vi "Main_VirtualAccelerometer.vi"() -> ()   [LabVIEW 2019]
panel:
  out "Pos RSQ":dbl
  out "Original Pos versus Accelerometer Double Integration":cluster{i32[], dbl[]}(graph)
  out "V. Accel":dbl(graph)
  out "Mouse X Abs":i32
  in  "b":dbl=0.005 format="%#_13g"
  in  "m":dbl=0.001 format="%#_13g"
  in  "k":dbl=2000.0 format="%#_13g"
  out "Spring and Mass Position":cluster{"Mouse X Abs":i32, "yk":dbl}[](graph)
  out "Spring and Mass Position":cluster{"Mouse X Abs":i32, "yk":dbl}(graph)
  in  "stop":bool
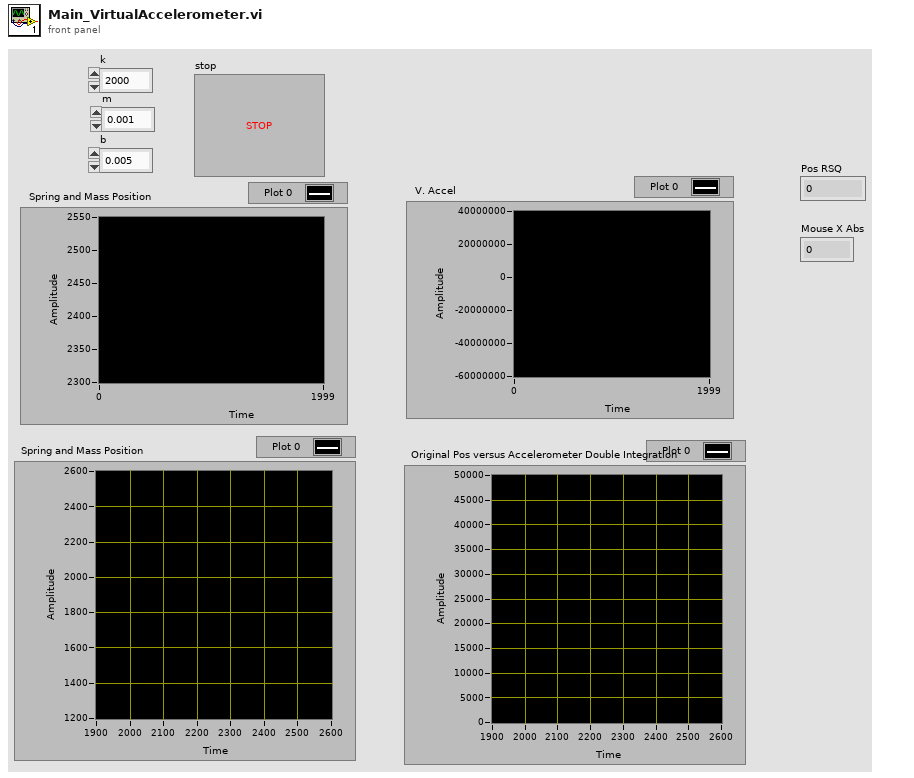
[diagram p1: front panel]
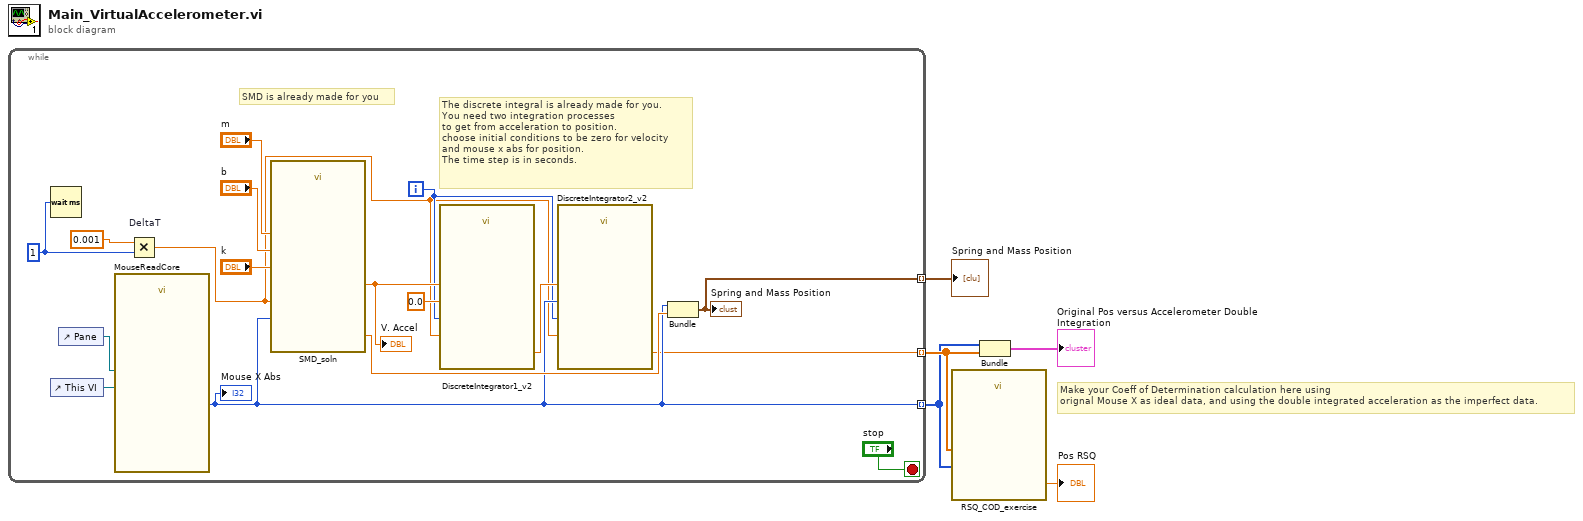
[diagram p0: block diagram]
diagram:
  # "Make your Coeff of Determination calculation here using\norignal Mouse X as ideal data, and using the double integrated acceleration as the imperfect data."
  n1 = while {
    tunnel: [w19] -> w5 mode=indexing
    tunnel: [w9] -> w1 mode=indexing
    tunnel: [w6] -> w2 mode=indexing
    i -> [w8]
    stop <- "stop" stop-if-true
    w13 = u32 1 ("milliseconds to wait")
    # "The discrete integral is already made for you.\nYou need two integration processes\nto get from acceleration to position.\nchoose initial conditions to be zero for velocity \nand mouse x abs for position.\nThe time step is in seconds."
    # "SMD is already made for you"
    n2 = Wait (ms)(milliseconds to wait=w13) -> ()  [unwired: 1 out]
    n3 = control-ref of="This VI"() -> (w21:refnum<vi>)
    n4 = control-ref of="Pane"() -> (w20:refnum<vi>)
    n5 = call "MouseReadCore.vi"("Pane"=w20, "VI in"=w21) -> ("Mouse X Abs"=w9:i32)  [unwired: 4 in, 5 out]
    "Mouse X Abs" <- w9
    n6 = Multiply "DeltaT"(x=0.001, y=w13) -> (x*y=w7:dbl)
    n7 = call "SMD_soln.vi"("k"="k", "b"="b", "m"="m", "Time Step"=w7, "xk"=w9) -> ("yk"=w15:dbl, "Accel"=w11:dbl)  [unwired: 5 in]
    "V. Accel" <- w11
    n8 = call "DiscreteIntegrator1_v2.vi"("Loop Iteration"=w8, "IC"=0.0, "Time Step"=w7, "Data in"=w11) -> ("Integ. Signal"=w10:dbl)  [unwired: 7 in]
    n9 = call "DiscreteIntegrator2_v2.vi"("Loop Iteration"=w8, "IC"=w9, "Time Step"=w7, "Data in"=w10) -> ("Integ. Signal"=w6:dbl)  [unwired: 7 in]
    n10 = Bundle("Mouse X Abs"=w9, "yk"=w15) -> (w19:cluster{"Mouse X Abs":i32, "yk":dbl})  [unwired: 1 in]
    "Spring and Mass Position" <- w19
  }
  "Spring and Mass Position" <- w5
  n11 = call "RSQ_COD_exercise.vi"("Data Yi's"=w2, "Model fi's"=w1) -> ("COD-RSQ"=→"Pos RSQ":dbl)  [unwired: 9 in]
  n12 = Bundle(w1, w2) -> (→"Original Pos versus Accelerometer Double Integration":cluster{i32[], dbl[]})  [unwired: 1 in]
